vi "Wait on Caller Idle.vi"(4 "ExecAnchor in":refnum<class "ExecAnchor.lvclass">) -> (1 "error out":errorcluster)   [LabVIEW 2020, in "ExecAnchor.lvclass"]
uses:
  ExecAnchor.lvclass
  ExecAnchor.lvclass/ExecAnchor.ctl
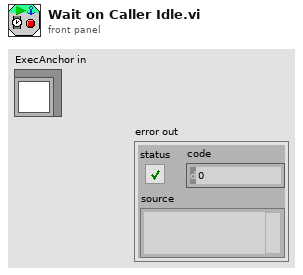
[diagram p1: front panel]
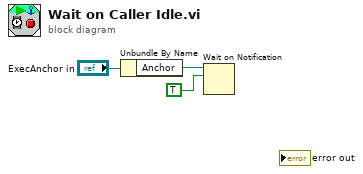
[diagram p0: block diagram]
diagram:
  n1 = Unbundle By Name("ExecAnchor in") -> ("Anchor"=w2:refnum<notifier>)
  n2 = Wait on Notification(notifier=w2, ignore previous (F)=TRUE) -> ()  [unwired: 2 in, 4 out]
